vi "LvMPDC_SUB_FindAtMusicFilePath_FileInfoDB.vi"(9 "file info[]":T2(array[cluster]) {"MusicInfo"."time" format="%<%H:%M:%S%3u>t"}, 11 "musicfile path":path) -> (0 "index":i32, 2 "MusicInfo":T1 {"time" format="%<%H:%M:%S%3u>t"})   [LabVIEW 2012]
uses:
  LvMPDC_Typdef_MusicInfo.ctl
panel:
  # "musicfile path と同じパスを持つものを、fileinfo[] から検索する - playlist で取得した filepath に該当する Title や Artist を取得するのに使う。"
  # "見つからなかったら(-1)を返す。"
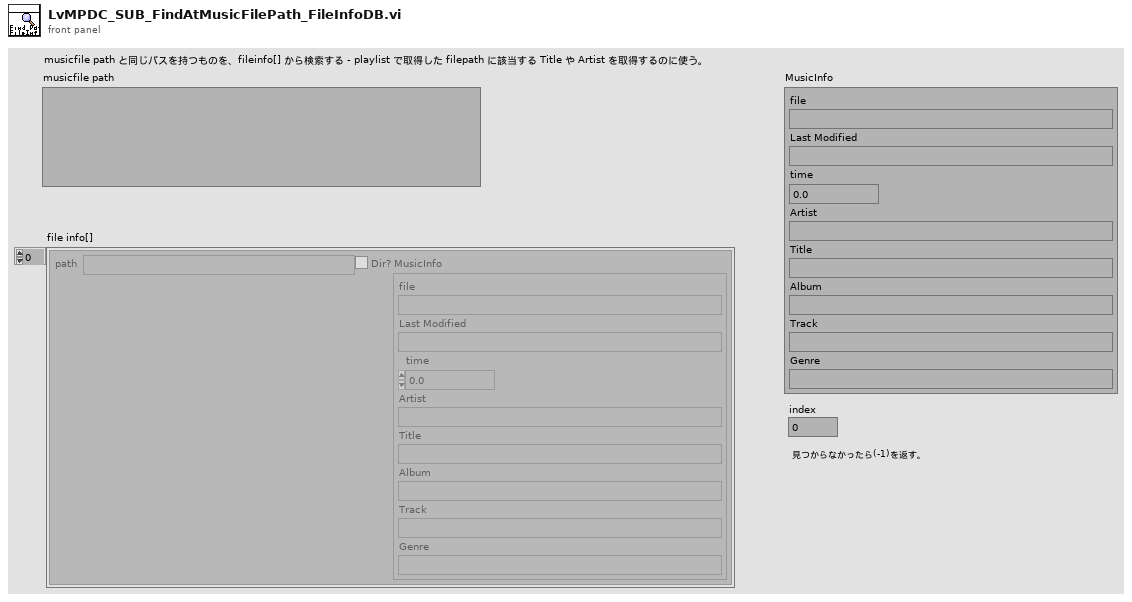
[diagram p1: front panel]
types:
  T1 = typedef "LvMPDC_Typdef_MusicInfo.ctl" = cluster{"file":string, "Last Modified":string, "time":dbl, "Artist":string, "Title":string, "Album":string, "Track":string, "Genre":string}
  T2 = cluster{"path":path, "Dir?":bool, "MusicInfo":T1}[]
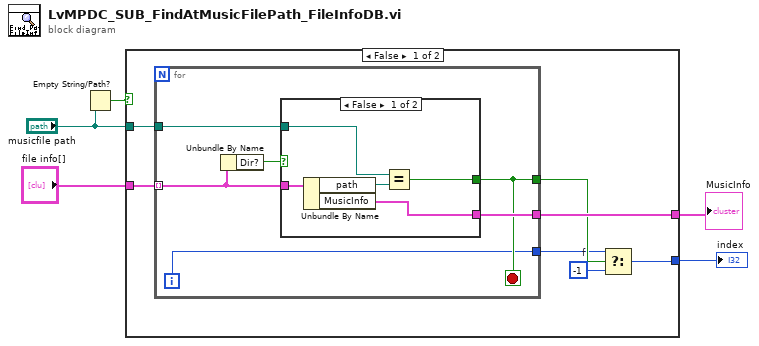
[diagram p0: block diagram]
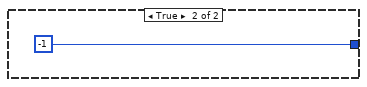
[diagram p3: hidden frame]
diagram:
  n1 = Empty String/Path?(string/path="musicfile path") -> (empty?=w2:bool)
  n2 = case shown="FALSE" w2 {
    tunnel: "file info[]" -> [w12 _]
    tunnel: "musicfile path" -> [w11 _]
    tunnel: [w10 _] -> w4
    tunnel: [w6 -1] -> w3
    frame False {
      w7 = -1  # f
      n3 = for {
        tunnel: w12 -> [w18] mode=indexing
        tunnel: w11 -> [w16]
        tunnel: [w15] -> w10
        tunnel: [w14] -> w9
        tunnel: [w13] -> w8
        i -> [w13]
        stop <- w14 stop-if-true
        n4 = Unbundle By Name(w18) -> ("Dir?"=w17:bool)
        n5 = case shown="FALSE" w17 {
          tunnel: w18 -> [w20 _]
          tunnel: w16 -> [w23 _]
          tunnel: [w21 _] -> w14
          tunnel: [w19 _] -> w15
          frame False {
            n6 = Unbundle By Name(w20) -> ("path"=w22:path, "MusicInfo"=w19:T1)
            n7 = Equal?(x=w23, y=w22) -> (x = y?=w21:bool)
          }
          frame True {
          }
        }
      }
      n8 = Select(t=w8, s=w9, f=w7) -> (s? t:f=w6:i32)
    }
    frame True {
    }
  }
  "MusicInfo" <- w4
  "index" <- w3
